vi "AverageBooleanValueOverTime.vi"(7 "input boolean":bool, 11 "sizeOfAverageArray (5)":i32=5) -> (8 "averaged":bool)   [LabVIEW 2020]
panel:
  out "array of values":i32[](array[numeric])
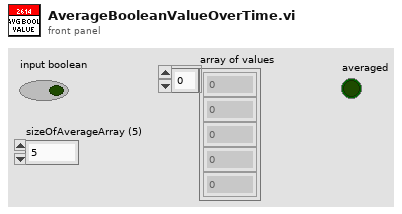
[diagram p1: front panel]
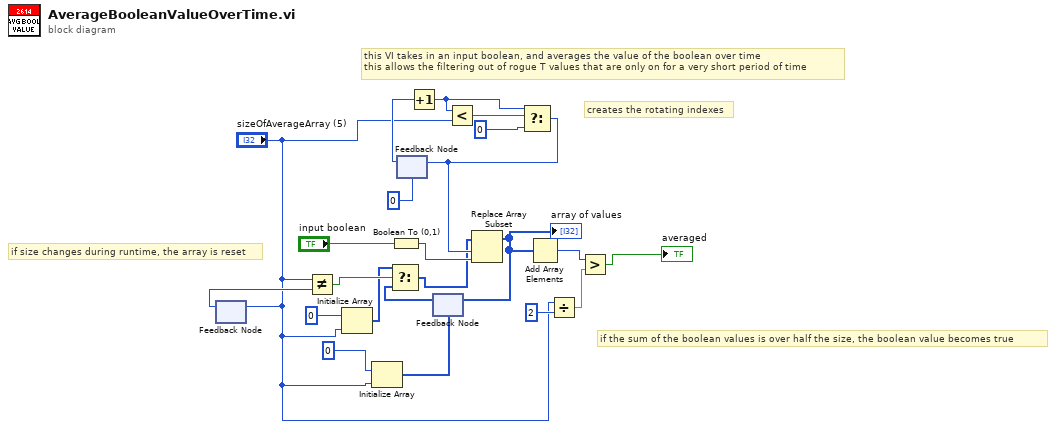
[diagram p0: block diagram]
diagram:
  # "if the sum of the boolean values is over half the size, the boolean value becomes true"
  # "creates the rotating indexes"
  # "if size changes during runtime, the array is reset"
  # "this VI takes in an input boolean, and averages the value of the boolean over time\nthis allows the filtering out of rogue T values that are only on for a very short period of time"
  n1 = feedback #1() -> (w6:i32)  [unwired: 1 in]
  n2 = feedback-in #1("sizeOfAverageArray (5)") -> ()
  n3 = Not Equal?(x="sizeOfAverageArray (5)", y=w6) -> (x != y?=w4:bool)
  n4 = Initialize Array(0, "sizeOfAverageArray (5)") -> (w2:i32[])
  n5 = Initialize Array(0, "sizeOfAverageArray (5)") -> (w20:i32[])
  n6 = Boolean To (0,1)(Boolean="input boolean") -> (0, 1=w19:i16)
  n7 = feedback #2(0) -> (w16:i32)
  n8 = Increment(x=w16) -> (x+1=w14:i32)
  n9 = feedback #3(w20) -> (w18:i32[])
  n10 = Select(t=w2, s=w4, f=w18) -> (s? t:f=w5:i32[])
  n11 = Less?(x=w14, y="sizeOfAverageArray (5)") -> (x < y?=w7:bool)
  n12 = Select(t=w14, s=w7, f=0) -> (s? t:f=w13:i32)
  n13 = feedback-in #2(w13) -> ()
  n14 = Replace Array Subset(array=w5, new element=w19, index=w13) -> (w12:i32[])
  "array of values" <- w12
  n15 = feedback-in #3(w12) -> ()
  n16 = Add Array Elements(numeric array=w12) -> (sum=w11:i32)
  n17 = Divide(x="sizeOfAverageArray (5)", y=2) -> (x/y=w9:dbl)
  n18 = Greater?(x=w11, y=w9) -> (0:→"averaged":bool)
